vi "Parse Frame Array File.vi"(8 "error in":errorcluster, 11 "frame array path in":path caption="path to parameters xml") -> (0 "error out":errorcluster, 2 "Frame Map array":T1[](array[typedef]) {"Data" format="%.0x"; "HeaderInfo"."NetSelect" items=["FDX_TX_FRAME_DLY_A"=0, "FDX_TX_FRAME_DLY_B"=1, "FDX_TX_FRAME_BOTH "=3, "FDX_TX_FRAME_ONLY_A"=4, "FDX_TX_FRAME_ONLY_B "=5]; "HeaderInfo"."FrameStartMode" items=["FDX_TX_FRAME_START_IFG", "FDX_TX_FRAME_START_PGWT", "FDX_TX_FRAME_START_TRG"]; "HeaderInfo"."PhysErrorInjection" items=["FDX_TX_FRAME_ERR_OFF"=0, "FDX_TX_FRAME_ERR_CRC"=1, "FDX_TX_FRAME_ERR_ALI"=2, "FDX_TX_FRAME_ERR_PRE"=4, "FDX_TX_FRAME_ERR_PHY"=8]; "HeaderInfo"."SequenceNumberInit" items=["FDX_TX_FRAME_SEQ_INIT_AUTO"=65535]; "HeaderInfo"."SequenceNumberOffset" items=["FDX_TX_FRAME_SEQ_OFFS_AUTO "=65535]; "HeaderInfo"."PayloadGenerationMode" items=["FDX_TX_FRAME_PGM_USER"=0, "FDX_TX_FRAME_PGM_IP_PART"=1, "FDX_TX_FRAME_PGM_IP_FULL"=2, "FDX_TX_FRAME_PGM_IP_PART_TT"=10, "FDX_TX_FRAME_PGM_IP_FULL_TT"=20]; "HeaderInfo"."PayloadBufferMode" items=["FDX_TX_FRAME_PBM_STD", "FDX_TX_FRAME_PBM_MAC", "FDX_TX_FRAME_PBM_UDP"]}, 3 "frame array path out":path caption="path to parameters xml")   [LabVIEW 2020, in "AIM ARINC 664 Scripting.lvlib"]
uses:
  AIM ARINC 664 Scripting.lvlib
  Frame Configuration/controls/frame_record_type.ctl
  <instrlib>/AIM GmbH/_AIM 664/_controls/queue_header_generic.ctl
  Frame Configuration/controls/frame_file_entry.ctl
  <instrlib>/AIM GmbH/_AIM 664/AIM664LV.lvlib
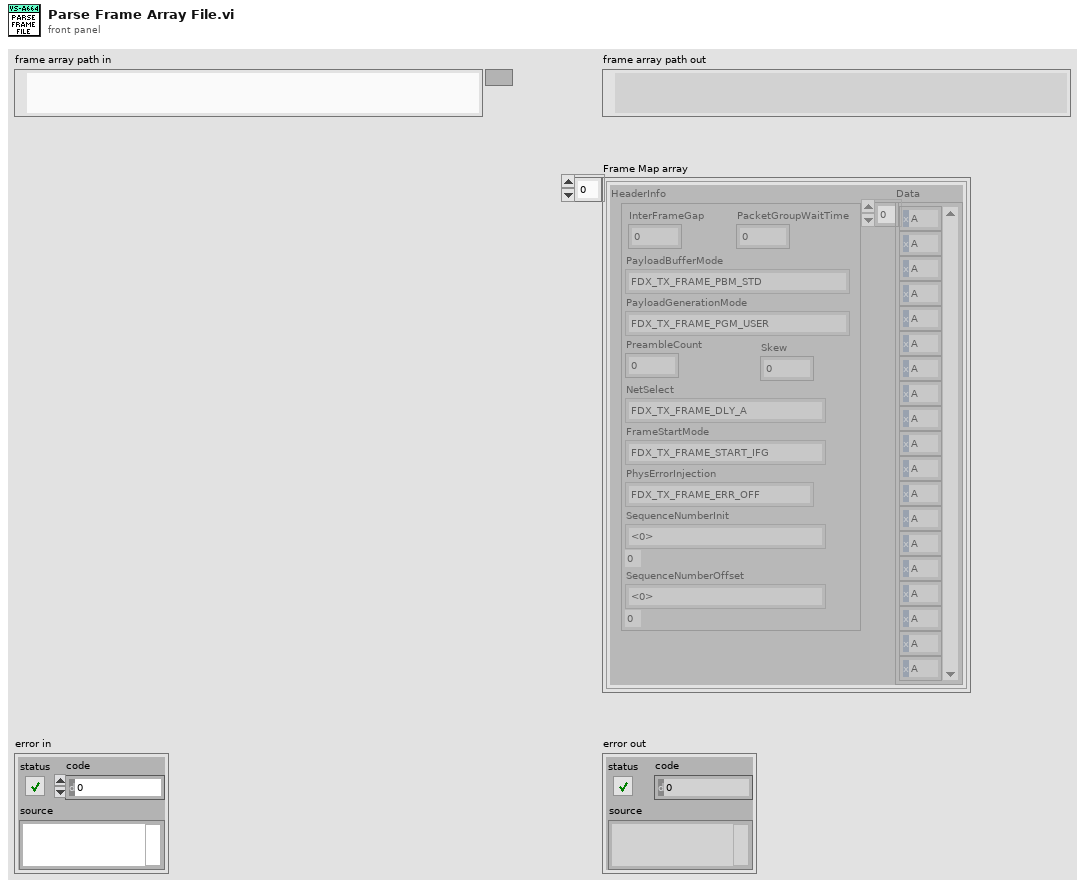
[diagram p1: front panel]
types:
  T1 = typedef "frame_record_type.ctl" = cluster{"HeaderInfo":T2, "Data":u8[]}
  T2 = typedef "AIM664LV.lvlib/queue_header_generic.ctl" = cluster{"InterFrameGap":u32, "PacketGroupWaitTime":u32, "PayloadBufferMode":u8, "PayloadGenerationMode":u8, "PreambleCount":u8, "Skew":u32, "NetSelect":u8, "FrameStartMode":u8, "PhysErrorInjection":u32, "SequenceNumberInit":u16, "SequenceNumberOffset":u16}
  T3 = typedef "frame_file_entry.ctl" = cluster{"key":string, "value":T1}
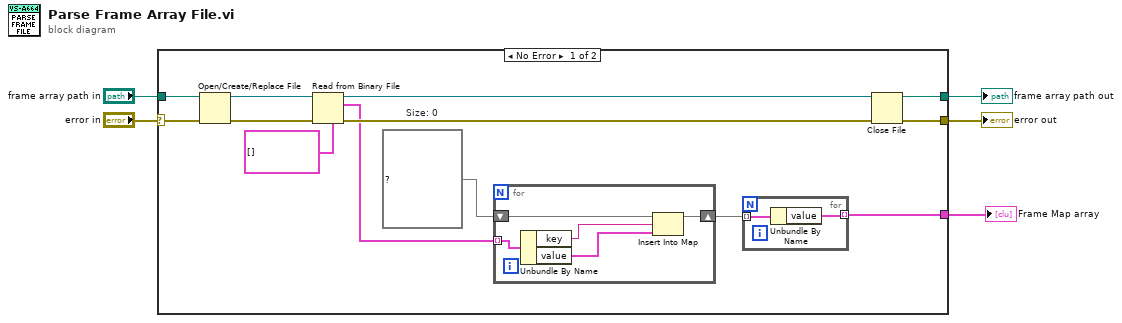
[diagram p0: block diagram]
diagram:
  n1 = case shown="No Error" "error in" {
    selector: "error in" -> [w8 w27]
    tunnel: [w9 w27] -> w5
    tunnel: "frame array path in" -> [w11 w26]
    tunnel: [w10 w26] -> w2
    tunnel: [w6 _] -> w1
    frame No Error {
      w18 = map{string, T1} {}  # Size: 0
      n2 = Open/Create/Replace File(file path (use dialog)=w11, error in=w8) -> (refnum out=w13:refnum<file>, error out=w17:errorcluster)  [unwired: 4 in, 1 out]
      n3 = Read from Binary File(5:T3[] [] ("cluster"), 8:w17, 11:w13) -> (0:w16:errorcluster, 2:w15:T3[], 3:w12:refnum<file>)  [unwired: 3 in, 1 out]
      n4 = for {
        shift-right: [w24] -> w7
        shift-left: w18 -> [w25]
        tunnel: w15 -> [w21] mode=indexing
        n5 = Unbundle By Name(w21) -> ("key"=w23:string, "value"=w22:T1)
        n6 = Insert Into Map(map in=w25, key=w23, value=w22) -> (map out=w24:map{string, T1})  [unwired: 2 out]
      }
      n7 = for {
        tunnel: w7 -> [w20] mode=indexing
        tunnel: [w19] -> w6 mode=indexing
        n8 = Unbundle By Name(w20) -> ("value"=w19:T1)
      }
      n9 = Close File(refnum=w12, error in=w16) -> (path=w10:path, error out=w9:errorcluster)
    }
    frame Error {
    }
  }
  "error out" <- w5
  "frame array path out" <- w2
  "Frame Map array" <- w1
